vi "createBroadcastFreezeForceFrame.vi"(8 "error in (no error)":errorcluster, 9 "TriggerIRQ":bool, 10 "WaitForTrigger":bool, 11 "FAILC in":refnum<class "FAILC.lvclass">) -> (0 "error out":errorcluster, 2 "Frame":T1 {"Data" format="%02x"}, 3 "FAILC out":refnum<class "FAILC.lvclass">)   [LabVIEW 2015, in "RTFAILC.lvlib" / "FAILC.lvclass"]
uses:
  FAILC.lvclass
  Common_RT_Modbus/DataTypes/Frame.ctl
  Common_RT_Modbus/DynamicFrameBuilder/DynamicFrameBuilder.lvclass
  Common_RT_Modbus/RTModbus.lvlib
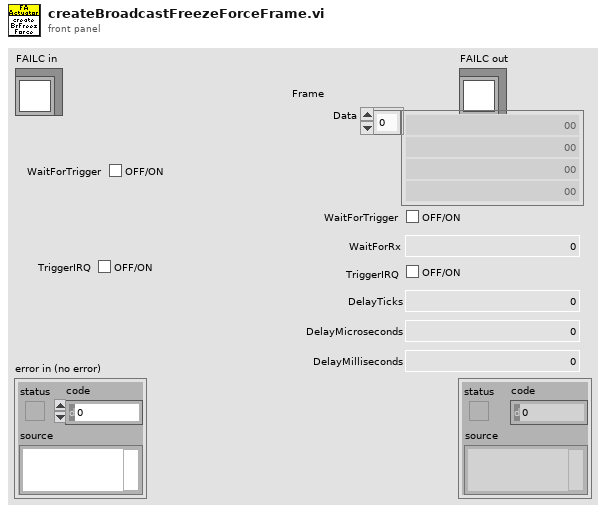
[diagram p1: front panel]
types:
  T1 = typedef "RTModbus.lvlib/Frame.ctl" = cluster{"Data":u8[], "WaitForTrigger":bool, "WaitForRx":u16, "TriggerIRQ":bool, "DelayTicks":u16, "DelayMicroseconds":u16, "DelayMilliseconds":u16}
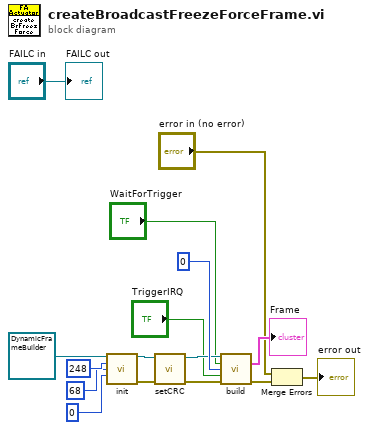
[diagram p0: block diagram]
diagram:
  n1 = call "init.vi"("DynamicFrameBuilder in"=refnum<class "DynamicFrameBuilder.lvclass"> refnum ("RTModbus.lvlib:DynamicFrameBuilder.lvclass"), "Address"=u8 248, "Function"=u8 68, "DataSize"=0) -> ("DynamicFrameBuilder out"=w15:refnum<class "DynamicFrameBuilder.lvclass">, "error out"=w14:errorcluster)  [unwired: 10 in]
  n2 = call "setCRC.vi"("error in (no error)"=w14, "DynamicFrameBuilder in"=w15) -> ("error out"=w12:errorcluster, "DynamicFrameBuilder out"=w11:refnum<class "DynamicFrameBuilder.lvclass">)  [unwired: 8 in]
  n3 = call "build.vi"("DynamicFrameBuilder in"=w11, "WaitForTrigger"="WaitForTrigger", "WaitForRxTimeout"=u16 0, "TriggerIRQ"="TriggerIRQ", "error in (no error)"=w12) -> ("Frame"=→"Frame":T1, "error out"=w3:errorcluster)  [unwired: 8 in, 1 out]
  n4 = Merge Errors("error in (no error)", w3) -> (→"error out":errorcluster)
  "FAILC out" <- "FAILC in"
